vi "Switch Window State.vi"(8 "error in (no error)":errorcluster, 10 "Enable (T)":bool=TRUE, 11 "Window VI's Ref":refnum<vi>) -> (0 "error out":errorcluster)   [LabVIEW 2013]
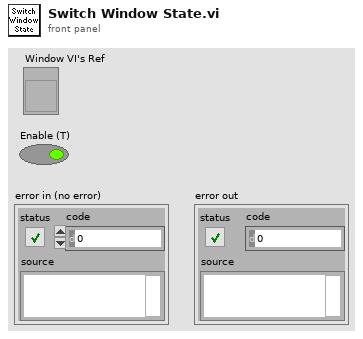
[diagram p1: front panel]
types:
  T1 = enum32{"Invalid", "Standard", "Closed", "Hidden", "Minimized", "Maximized"}
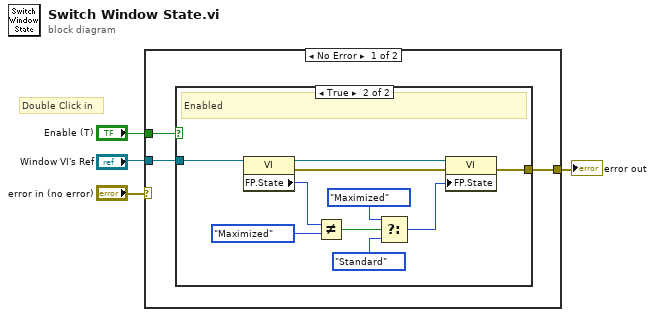
[diagram p0: block diagram]
diagram:
  # "Double Click in"
  n1 = case shown="No Error" "error in (no error)" {
    selector: "error in (no error)" -> [_ w18]
    tunnel: "Enable (T)" -> [w7 _]
    tunnel: "Window VI's Ref" -> [w6 _]
    tunnel: [w5 w18] -> w2
    frame No Error {
      n2 = case shown="True" w7 {
        tunnel: w6 -> [_ w10]
        tunnel: [_ w8] -> w5
        frame False {
          # "Disabled"
        }
        frame True {
          # "Enabled"
          n3 = property class="VI"(reference=w10) -> (reference out=w17:refnum<vi>, error out=w9:errorcluster, "FP.State"=w12:T1)  [unwired: 1 in]
          n4 = Not Equal?(x=w12, y=T1."Maximized" ("Front Panel Window:State")) -> (x != y?=w13:bool)
          n5 = Select(t=T1."Maximized" ("Front Panel Window:State"), s=w13, f=T1."Standard" ("Front Panel Window:State")) -> (s? t:f=w16:T1)
          n6 = property class="VI"(reference=w17, error in=w9, "FP.State"=w16) -> (error out=w8:errorcluster)  [unwired: 1 out]
        }
      }
    }
    frame Error {
    }
  }
  "error out" <- w2
